vi "calculator 1.vi"() -> ()   [LabVIEW 2017]
panel:
  out "Result":dbl
  in  "Select":enum16{"add", "sub", "multiply", "divide"}(ring)
  in  "Numeric 2":dbl
  in  "Numeric 1":dbl
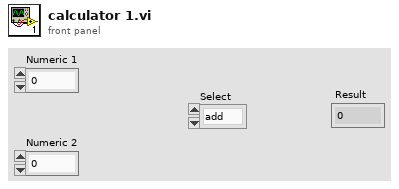
[diagram p1: front panel]
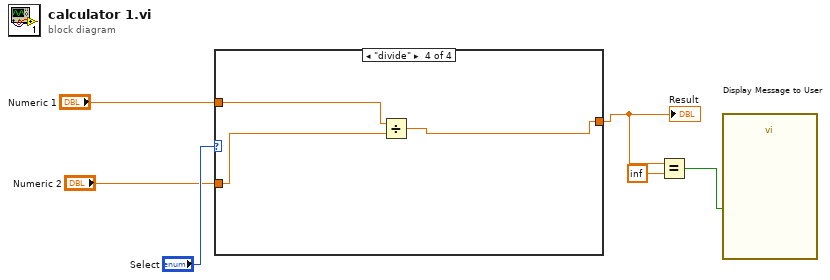
[diagram p0: block diagram]
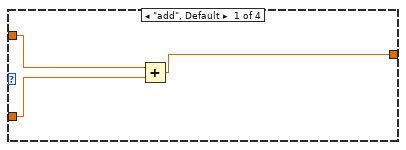
[diagram p2: hidden frame]
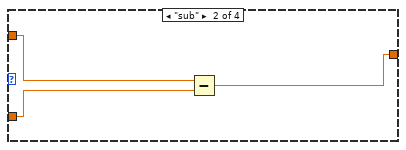
[diagram p3: hidden frame]
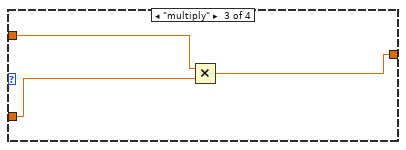
[diagram p4: hidden frame]
diagram:
  n1 = case shown="\"divide\"" "Select" {
    tunnel: "Numeric 1" -> [w9 w12 w15 w16]
    tunnel: "Numeric 2" -> [w8 w11 w14 w18]
    tunnel: [w7 w10 w13 w17] -> w3
    frame "add", Default {
      n2 = Add(x=w9, y=w8) -> (x+y=w7:dbl)
    }
    frame "sub" {
      n3 = Subtract(x=w12, y=w11) -> (x-y=w10:dbl)
    }
    frame "multiply" {
      n4 = Multiply(x=w15, y=w14) -> (x*y=w13:dbl)
    }
    frame "divide" {
      n5 = Divide(x=w16, y=w18) -> (x/y=w17:dbl)
    }
  }
  "Result" <- w3
  n6 = Equal?(x=w3, y=inf) -> (x = y?=w1:bool)
  n7 = call "Display Message to User"("Enable"=w1) -> ()  [unwired: 9 in, 2 out]
